vi "Write ADU Packet.vi"(8 "error in":errorcluster, 9 "modbus data unit":refnum<class "Modbus Data Unit.lvclass">, 10 "protocol layer":refnum<class "Network Protocol.lvclass">, 11 "RTU transmission data unit in":refnum<class "RTU Data Unit.lvclass">) -> (0 "error out":errorcluster, 2 "protocol layer out":refnum<class "Network Protocol.lvclass">, 3 "RTU transmission data unit out":refnum<class "RTU Data Unit.lvclass">)   [LabVIEW 2012, in "RTU Data Unit.lvclass"]
uses:
  RTU Data Unit.lvclass
  Modbus Data Unit/Modbus Data Unit.lvclass
  Network Protocol/Network Protocol.lvclass
  Modbus Data Unit/Modbus Data Unit.lvclass/Modbus Data Unit.ctl
  Serial Interface/Serial Data Unit.lvclass/Serial Data Unit.ctl
  Transmission Data Unit.lvclass/Transmission Data Unit.ctl
  <vilib>/Utility/error.llb/Error Cluster From Error Code.vi
  <vilib>/ErrorRing/Error Ring.xnode
  Transmission Data Unit.lvclass
  Serial Interface/Serial Data Unit.lvclass
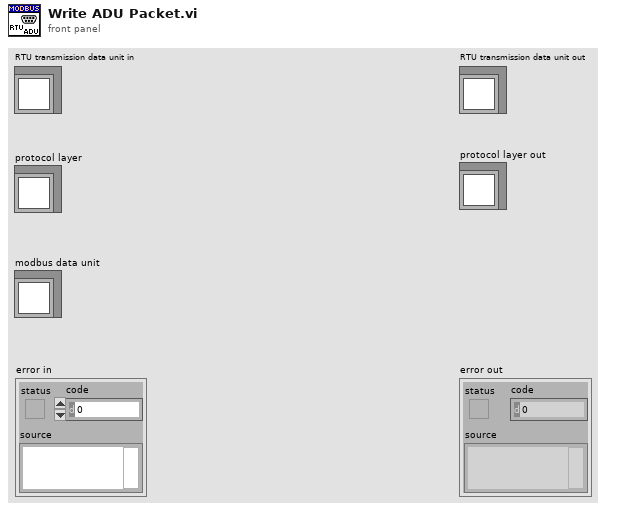
[diagram p1: front panel]
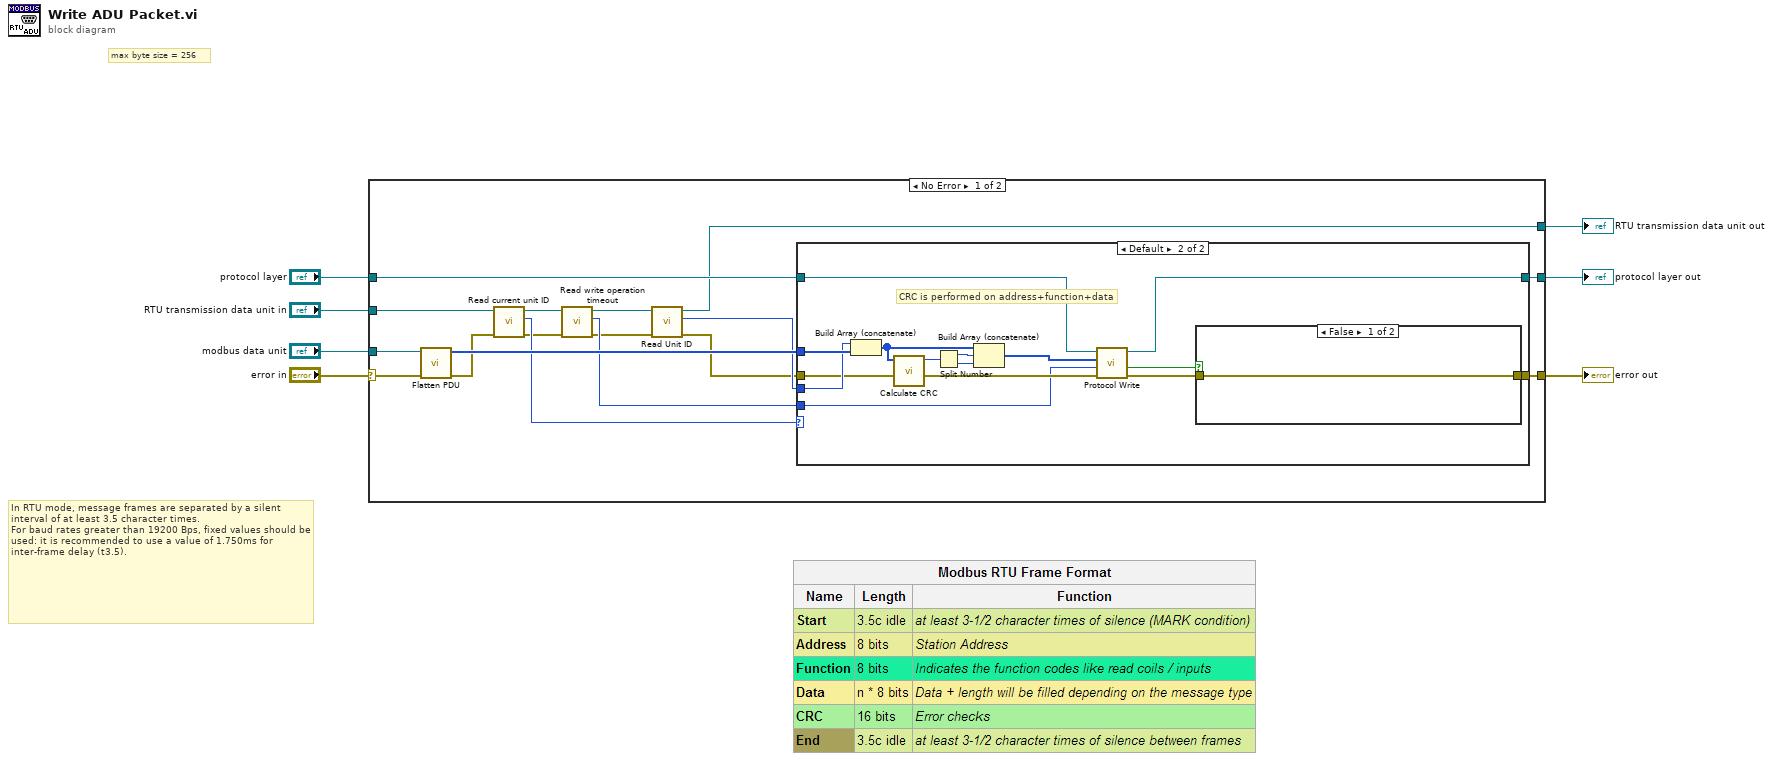
[diagram p0: block diagram]
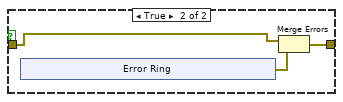
[diagram p3: hidden frame]
diagram:
  # "max byte size = 256"
  # "In RTU mode, message frames are separated by a silent interval of at least 3.5 character times.\nFor baud rates greater than 19200 Bps, fixed values should be used: it is recommended to use a value of 1.750ms for inter-frame delay (t3.5)."
  n1 = case shown="No Error" "error in" {
    selector: "error in" -> [w19 w51]
    tunnel: [w20 w51] -> w6
    tunnel: "modbus data unit" -> [w24 _]
    tunnel: "RTU transmission data unit in" -> [w12 w49]
    tunnel: "protocol layer" -> [w22 w50]
    tunnel: [w21 w50] -> w1
    tunnel: [w14 w49] -> w2
    frame No Error {
      n2 = call "Flatten PDU.vi"("error in"=w19, "modbus data unit in"=w24) -> ("error out"=w13:errorcluster, "Full modbus data unit"=w23:u8[])  [unwired: 8 in]
      n3 = call "Read current unit ID.vi"("error in (no error)"=w13, "Serial Data Unit in"=w12) -> ("error out"=w8:errorcluster, "request unit ID"=w18:u8, "Serial Data Unit out"=w11:refnum<class "RTU Data Unit.lvclass">)  [unwired: 7 in]
      n4 = call "Read write operation timeout.vi"("error in (no error)"=w8, "transmission data unit in"=w11) -> ("error out"=w9:errorcluster, "write operation timeout"=w17:i32, "transmission data unit out"=w10:refnum<class "RTU Data Unit.lvclass">)  [unwired: 7 in]
      n5 = call "Read Unit ID.vi"("error in"=w9, "transmission data unit in"=w10) -> ("error out"=w15:errorcluster, "unit ID"=w16:u8, "transmission data unit out"=w14:refnum<class "RTU Data Unit.lvclass">)  [unwired: 7 in]
      n6 = case shown="Default" w18 {
        tunnel: w23 -> [_ w40]
        tunnel: w16 -> [_ w39]
        tunnel: w15 -> [w26 w38]
        tunnel: w22 -> [w25 w37]
        tunnel: [w25 w36] -> w21
        tunnel: [w26 w28] -> w20
        tunnel: w17 -> [_ w27]
        frame 0 {
          # "request unit ID defaults to 1. If it is 0 it was set that way. If it was set that way, this is a slave trying to respond to a broadcast"
        }
        frame Default {
          # "CRC is performed on address+function+data"
          n7 = Build Array (concatenate)(w39, w40) -> (w35:u8[])
          n8 = call "Calculate CRC.vi"("data"=w35) -> ("CRC-16"=w33:u16)  [unwired: 10 in]
          n9 = Split Number(x=w33) -> (hi(x)=w32:u8, lo(x)=w31:u8)
          n10 = Build Array (concatenate)(w35, w32, w31) -> (w34:u8[])
          n11 = call-dynamic "Protocol Write.vi"("error in"=w38, "timeout"=w27, "data"=w34, "protocol layer in"=w37) -> ("error out"=w29:errorcluster, "timed out?"=w30:bool, "protocol layer out"=w36:refnum<class "Network Protocol.lvclass">)  [unwired: 5 in]
          n12 = case shown="False" w30 {
            tunnel: w29 -> [w41 w43]
            tunnel: [w41 w44] -> w28
            frame False {
            }
            frame True {
              n13 = xnode "Error Ring"() -> ("error out"=w42:errorcluster)
              n14 = Merge Errors(w43, w42) -> (w44:errorcluster)
            }
          }
        }
      }
    }
    frame Error {
    }
  }
  "error out" <- w6
  "RTU transmission data unit out" <- w2
  "protocol layer out" <- w1
